vi "Example 2.vi"() -> ()   [LabVIEW 2016]
uses:
  listbox/listbox.lvclass
  LNK/Copy/Copy.lvclass
  C:/Users/ok/Desktop/ListboxMenu/LNK/Parent Class/Menu.lvclass
  LNK/Delete/Delete.lvclass
  LNK/UP/UP.lvclass
  LNK/Down/Down.lvclass
  listbox/listbox.lvclass/listbox.ctl
panel:
  in  "停止":bool
  in  "多列列表框":i32(listbox)=4
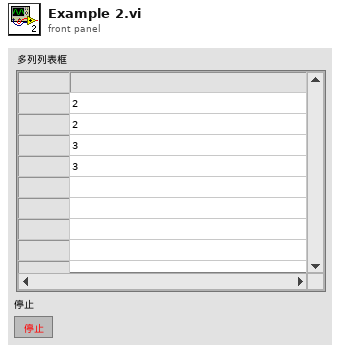
[diagram p1: front panel]
types:
  T1 = typedef "LVPoint32TypeDef.ctl" = cluster{"Horizontal":i32, "Vertical":i32}
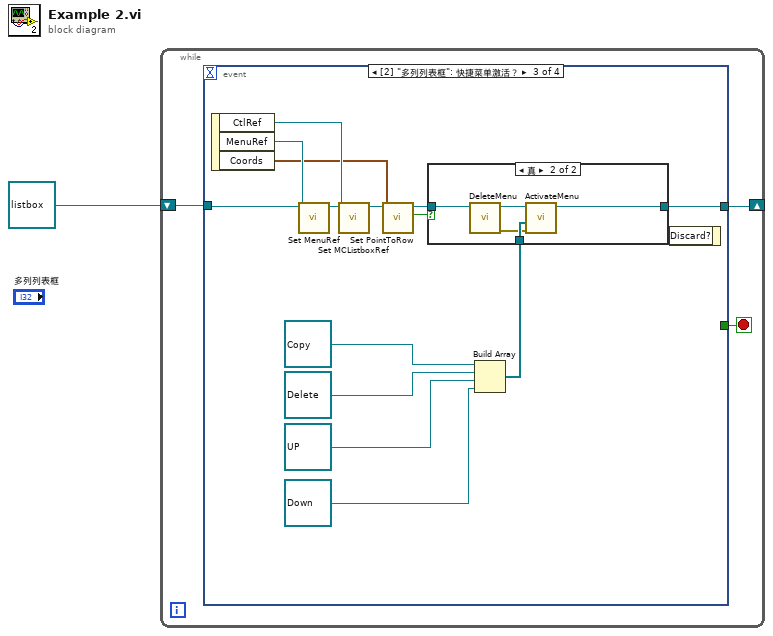
[diagram p0: block diagram]
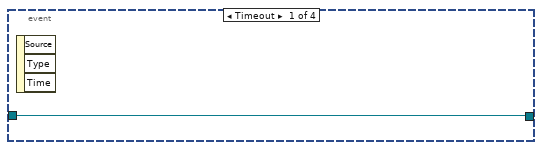
[diagram p2: hidden frame]
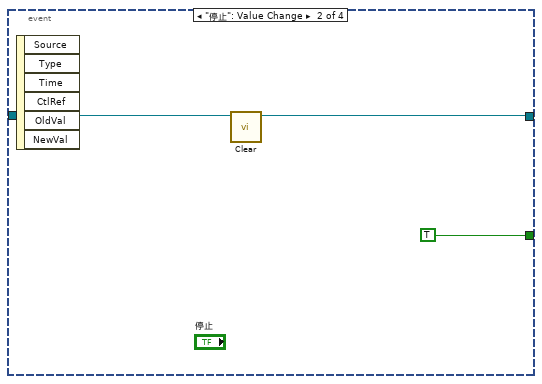
[diagram p3: hidden frame]
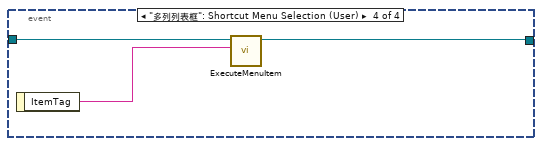
[diagram p5: hidden frame]
diagram:
  n1 = while {
    shift-right: [w2] -> _
    shift-left: refnum<class "listbox.lvclass"> refnum ("listbox.lvclass") -> [w3]
    stop <- w4 stop-if-true
    n2 = event shown="[2] \"多列列表框\": 快捷菜单激活？" {
      selector: _ -> [_ _ _ _]
      dyn-events: _ -> [_ _ _ _]
      timeout: _ -> [_ _ _ _]
      tunnel: [_ TRUE _ _] -> w4
      tunnel: w3 -> [w5 w7 w22 w31]
      tunnel: [w5 w6 w18 w30] -> w2
      event Timeout {
        n3 = event-data() -> ()  [unwired: 1 in, 3 out]
      }
      event "停止": Value Change {
        n4 = event-data() -> ()  [unwired: 1 in, 6 out]
        n5 = call "Clear.vi"("listbox 输入"=w7) -> ("listbox 输出"=w6:refnum<class "listbox.lvclass">)  [unwired: 9 in, 1 out]
      }
      event "多列列表框": Shortcut Menu Activation? {
        n6 = event-data() -> ("CtlRef"=w17:refnum<vi>, "MenuRef"=w21:refnum<k9>, "Coords"=w15:T1)  [unwired: 1 in]
        n7 = call "Set MenuRef.vi"("MenuRef"=w21, "listbox in"=w22) -> ("listbox out"=w20:refnum<class "listbox.lvclass">)  [unwired: 9 in]
        n8 = call "Set MCListboxRef.vi"("MCListboxRef"=w17, "listbox in"=w20) -> ("listbox out"=w19:refnum<class "listbox.lvclass">)  [unwired: 9 in]
        n9 = call "Set PointToRow.vi"("坐标"=w15, "listbox 输入"=w19) -> ("边界内？"=w14:bool, "listbox 输出"=w16:refnum<class "listbox.lvclass">)  [unwired: 7 in, 1 out]
        n10 = Build Array(refnum<class "Copy.lvclass"> refnum ("Copy.lvclass"), refnum<class "Delete.lvclass"> refnum ("Delete.lvclass"), refnum<class "UP.lvclass"> refnum ("UP.lvclass"), refnum<class "Down.lvclass"> refnum ("Down.lvclass")) -> (w11:refnum<class "Menu.lvclass">[])
        n11 = case shown="真" w14 {
          tunnel: w11 -> [_ w28]
          tunnel: [w23 w24] -> w18
          tunnel: w16 -> [w23 w25]
          frame False {
          }
          frame True {
            n12 = call "DeleteMenu.vi"("listbox 输入"=w25) -> ("error out"=w26:errorcluster, "listbox 输出"=w27:refnum<class "listbox.lvclass">)  [unwired: 9 in]
            n13 = call "ActivateMenu.vi"("error in (no error)"=w26, "MenuClassArray"=w28, "listbox 输入"=w27) -> ("listbox 输出"=w24:refnum<class "listbox.lvclass">)  [unwired: 7 in, 1 out]
          }
        }
        n14 = event-data() -> ()  [unwired: 2 in, 1 out]
      }
      event "多列列表框": Shortcut Menu Selection (User) {
        n15 = event-data() -> ("ItemTag"=w29:string)  [unwired: 1 in]
        n16 = call "ExecuteMenuItem.vi"("项标识符"=w29, "listbox 输入"=w31) -> ("listbox 输出"=w30:refnum<class "listbox.lvclass">)  [unwired: 8 in, 1 out]
      }
    }
  }
